vi "New.vi"(10 "config file":path, 11 "subhandler":refnum<class "Formatting Handler.lvclass">) -> (3 "test handler out":refnum<class "Test Handler.lvclass">)   [LabVIEW 2018, in "Test Handler.lvclass"]
uses:
  Test Handler.lvclass
  src/api/extension/formatting_handler_interface/Formatting Handler.lvclass
  Test Handler.lvclass/Test Handler.ctl
panel:
  # "Connector Pane"
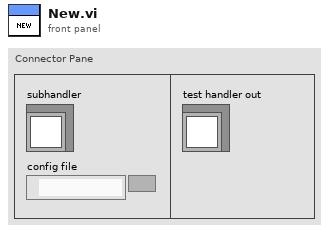
[diagram p1: front panel]
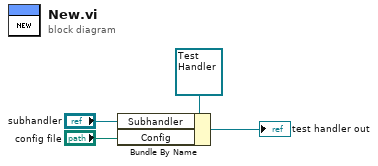
[diagram p0: block diagram]
diagram:
  n1 = Bundle By Name(cluster=refnum<class "Test Handler.lvclass"> refnum ("test handler in"), "Subhandler"="subhandler", "Config"="config file") -> (→"test handler out":refnum<class "Test Handler.lvclass">)
